vi "SigGen-Compute Max Level (full, arbitrary).vi"(0 "Level":T1, 1 "MinFreq":dbl, 2 "MaxFreq":dbl, 5 "Y":dbl[](array[numeric]), 7 "Sampling Rate (Hz)":dbl, 9 "Npts":i32, 11 "error in (no error)":errorcluster) -> (4 "Level Out":T1, 14 "Max Level":dbl, 15 "error out":errorcluster)   [LabVIEW 2020]
uses:
  Controls/Level XCtl/Level Data.ctl
  Controls/Level XCtl/Level Units.ctl
  <vilib>/Analysis/5stat.llb/RMS (DBL).vi
  PXI DAQ VIs/DAQ Engine VIs/PXI Globals.vi
  Utility VIs/Math VIs/Linear to dB (scalar).vi
  Utility VIs/Math VIs/FFT x(t) to dB,Degrees (1D).vi
  <vilib>/Analysis/NI_AALPro.lvlib
  Controls/Level XCtl/Level XCtl.xctl
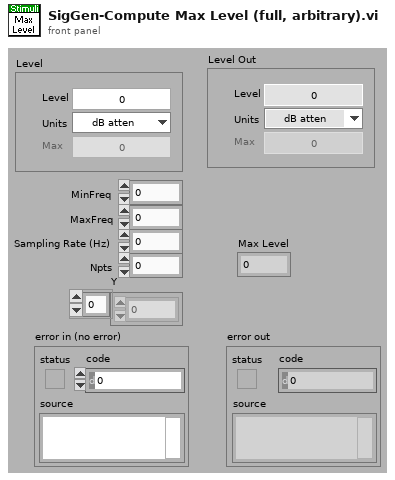
[diagram p1: front panel]
types:
  T1 = typedef "Level XCtl.xctl/Level Data.ctl" = cluster{"Level":dbl, "Units":T2, "Max":dbl, "Multiplier":dbl, "Cal File":path, "Cal":cluster{"Freq (Hz)":dbl[], "Mag (dB SPL)":dbl[], "Phase (deg)":dbl[]}}
  T2 = typedef "Level Units.ctl" = enum16{"dB atten", "dB SPL", "dB re 1 Vrms", "dB V/Hz½", "mW", "dB HL", "Volts", "dB mW"}
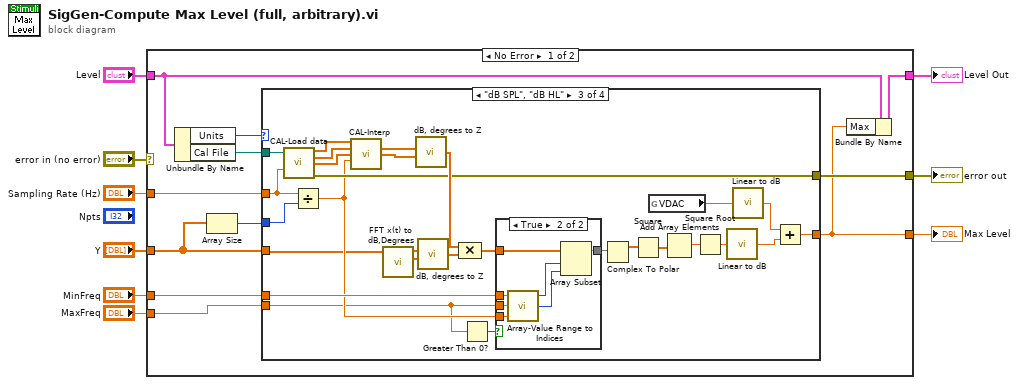
[diagram p0: block diagram]
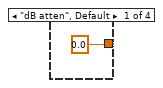
[diagram p2: hidden frame]
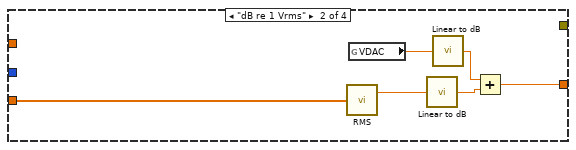
[diagram p3: hidden frame]
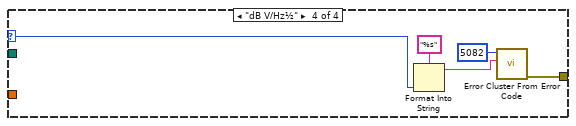
[diagram p5: hidden frame]
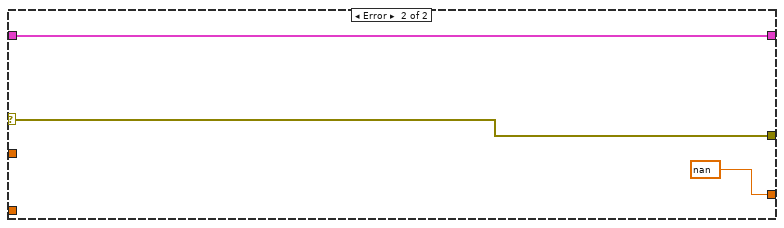
[diagram p6: hidden frame]
diagram:
  n1 = case shown="No Error" "error in (no error)" {
    selector: "error in (no error)" -> [_ w71]
    tunnel: "Level" -> [w19 w69]
    tunnel: [w20 w71] -> w7
    tunnel: [w18 nan ("Reference Level")] -> w9
    tunnel: [w17 w69] -> w6
    tunnel: "Y" -> [w13 _]
    tunnel: "Sampling Rate (Hz)" -> [w14 _]
    tunnel: "MinFreq" -> [w11 _]
    tunnel: "MaxFreq" -> [w10 _]
    frame No Error {
      n2 = Unbundle By Name(w19) -> ("Units"=w16:T2, "Cal File"=w15:path)
      n3 = Array Size(array=w13) -> (size(s)=w12:i32)
      n4 = case shown="\"dB SPL\", \"dB HL\"" w16 {
        selector: w16 -> [_ _ _ w64]
        tunnel: [0.0 ("Reference Level") w22 w54 _] -> w18
        tunnel: [_ _ w37 w65] -> w20
        tunnel: w15 -> [_ _ w52 _]
        tunnel: w13 -> [_ w27 w29 _]
        tunnel: w14 -> [_ _ w28 _]
        tunnel: w12 -> [_ _ w30 _]
        tunnel: w11 -> [_ _ w34 _]
        tunnel: w10 -> [_ _ w31 _]
        frame "dB atten", Default {
        }
        frame "dB re 1 Vrms" {
          n5 = call-poly <vilib>:"RMS.vi"("X"=w27) -> ("rms value"=w23:dbl)  [unwired: 1 out]
          n6 = global read "PXI Globals.vi" "VDAC"() -> (w26:dbl)
          n7 = call-poly "Linear to dB.vi"("Linear"=w23) -> ("dB"=w24:dbl)
          n8 = call-poly "Linear to dB.vi"("Linear"=w26) -> ("dB"=w25:dbl)
          n9 = Add(x=w25, y=w24) -> (x+y=w22:dbl)
        }
        frame "dB SPL", "dB HL" {
          n10 = call "CAL-Load data.vi"("user path"=w52, "Desired Fs (Hz)"=w28) -> ("Frequency (Hz)"=w49:dbl[], "Mag"=w48:dbl[], "Phase"=w47:dbl[], "error out"=w37:errorcluster)  [unwired: 6 in, 4 out]
          n11 = Divide(x=w28, y=w30) -> (x/y=w33:dbl)
          n12 = call "CAL-Interp.vi"("Frequency (Hz)"=w49, "Magnitude (dB)"=w48, "Phase (degrees)"=w47, "df (Hz)"=w33) -> ("Interp Magnitude (dB)"=w46:dbl[], "Interp Phase (degrees)"=w45:dbl[])  [unwired: 8 in, 2 out]
          n13 = call-poly "FFT x(t) to dB,Degrees.vi"("X"=w29) -> ("+Freq Phase of FFT (degrees)"=w43:dbl[], "+Freq. Mag of FFT (dB rms)"=w44:dbl[])  [unwired: 8 in, 1 out]
          n14 = call "dB, degrees to Z.vi"("Magnitude (dB)"=w46, "Phase (degrees)"=w45) -> ("Z"=w50:cdb[])  [unwired: 5 in]
          n15 = call "dB, degrees to Z.vi"("Magnitude (dB)"=w44, "Phase (degrees)"=w43) -> ("Z"=w36:cdb[])  [unwired: 5 in]
          n16 = Compound Arithmetic op=MULTIPLY(w50, w36) -> (w51:cdb[])
          n17 = Greater Than 0?(x=w31) -> (x > 0?=w32:bool)
          n18 = case shown="True" w32 {
            tunnel: w51 -> [w56 w63]
            tunnel: [w56 w62] -> w35
            tunnel: w34 -> [_ w59]
            tunnel: w31 -> [_ w58]
            tunnel: w33 -> [_ w57]
            frame False {
            }
            frame True {
              n19 = call "Array-Value Range to Indices.vi"("dx"=w57, "Xmax"=w58, "Xmin"=w59) -> ("Length"=w60:i32, "Offset"=w61:i32)  [unwired: 1 in]
              n20 = Array Subset(array=w63, index=w61, length=w60) -> (w62:cdb[])
            }
          }
          n21 = Complex To Polar(r * e^(i*theta)=w35) -> (r=w39:dbl[])  [unwired: 1 out]
          n22 = Square(x=w39) -> (x^2=w42:dbl[])
          n23 = global read "PXI Globals.vi" "VDAC"() -> (w55:dbl)
          n24 = Add Array Elements(numeric array=w42) -> (sum=w41:dbl)
          n25 = Square Root(x=w41) -> (sqrt(x)=w40:dbl)
          n26 = call-poly "Linear to dB.vi"("Linear"=w40) -> ("dB"=w38:dbl)
          n27 = call-poly "Linear to dB.vi"("Linear"=w55) -> ("dB"=w53:dbl)
          n28 = Add(x=w53, y=w38) -> (x+y=w54:dbl)
        }
        frame "dB V/Hz½" {
          n29 = Format Into String(format string="%s", w64) -> (resulting string=w67:string)  [unwired: 2 in, 1 out]
          n30 = call <vilib>:"Error Cluster From Error Code.vi"("error message (\"\")"=w67, "error code (0)"=5082) -> ("error out"=w65:errorcluster)  [unwired: 7 in]
        }
      }
      n31 = Bundle By Name(cluster=w19, "Max"=w18) -> (w17:T1)
    }
    frame Error {
    }
  }
  "error out" <- w7
  "Max Level" <- w9
  "Level Out" <- w6
